vi "Enqueue Data.vi"(8 "error in (no error)":errorcluster, 10 "Data":dbl, 11 "Test 1 in":refnum<class "Test 1.lvclass">) -> (0 "error out":errorcluster, 3 "Test 1 out":refnum<class "Test 1.lvclass">)   [LabVIEW 2022 SP3, in "Scratchpad.lvlib" / "Test 1.lvlib" / "Test 1.lvclass"]
uses:
  Test 1.lvclass
  Test 1.lvclass/Test 1.ctl
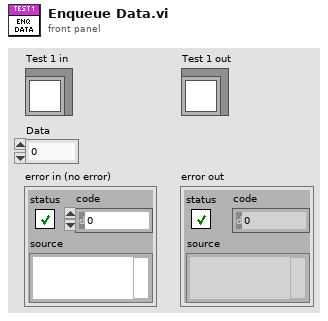
[diagram p1: front panel]
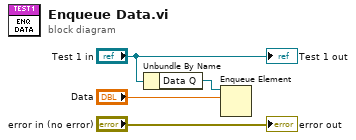
[diagram p0: block diagram]
diagram:
  n1 = Unbundle By Name("Test 1 in") -> ("Data Q"=w2:refnum<queue>)
  n2 = Enqueue Element(queue=w2, element="Data") -> ()  [unwired: 2 in, 3 out]
  "error out" <- "error in (no error)"
  "Test 1 out" <- "Test 1 in"
